vi "Structure Handler.vi"() -> ()   [LabVIEW 2010] (continued)
   .650136101028E-04   .693103789942E-04   .738911130024E-04   .787745775169E-04   .839807778292E-04\n   .895310410335E-04   .954481033336E-04   .101756203113E-03   .108481180149E-03   .115650581371E-03\n   .123293773602E-03   .131442063738E-03   .140128826854E-03   .149389642765E-03   .159262441590E-03\n   .169787658919E-03   .181008401214E-03   .192970622109E-03   .205723310339E-03   .219318690051E-03\n   .233812434316E-03   .249263892711E-03   .265736333886E-03   .283297204114E-03   .302018402857E-03\n   .321976576476E-03   .343253431267E-03   .365936067091E-03   .390117332948E-03   .415896205926E-03\n   .443378195057E-03   .472675771709E-03   .503908828239E-03   .537205166754E-03   .572701019950E-03\n   .610541606096E-03   .650881720414E-03   .693886365185E-03   .739731421127E-03   .788604362696E-03\n   .840705020160E-03   .896246391477E-03   .955455507177E-03   .101857435167E-02   .108586084462E-02\n   .115758988621E-02   .123405447041E-02   .131556687066E-02   .140245990241E-02   .149508826758E-02\n   .159382998615E-02   .169908792015E-02   .181129139623E-02   .193089793270E-02   .205839507779E-02\n   .219430236596E-02   .233917339963E-02   .249359806416E-02   .265820488411E-02   .283366352974E-02\n   .302068748250E-02   .322003686958E-02   .343252147732E-02   .365900395451E-02   .390040321649E-02\n   .415769806226E-02   .443193101665E-02   .472421241091E-02   .503572471499E-02   .536772713610E-02\n   .572156049811E-02   .609865241743E-02   .650052279140E-02   .692878961584E-02   .738517514896E-02\n   .787151243951E-02   .838975223731E-02   .894197030486E-02   .953037514915E-02   .101573161929E-01\n   .108252924048E-01   .115369614078E-01   .122951490860E-01   .131028597072E-01   .139632865812E-01\n   .148798232710E-01   .158560753728E-01   .168958728802E-01   .180032831452E-01   .191826244469E-01\n   .204384801745E-01   .217757136292E-01   .231994834433E-01   .247152596108E-01   .263288401171E-01\n   .280463681475E-01   .298743498448E-01   .318196725793E-01   .338896236775E-01   .360919095467E-01\n   .384346751137E-01   .409265234803E-01   .435765356742E-01   .463942903543E-01   .493898832987E-01\n   .525739464755E-01   .559576664626E-01   .595528019418E-01   .633716999509E-01   .674273105302E-01\n   .717331993426E-01   .763035577917E-01   .811532100904E-01   .862976166680E-01   .917528732159E-01\n   .975357045937E-01   .103663452719E+00   .110154057471E+00   .117026029513E+00   .124298413867E+00\n   .131990742895E+00   .140122977286E+00   .148715433467E+00   .157788695785E+00   .167363511634E+00\n   .177460667645E+00   .188100844913E+00   .199304451187E+00   .211091427879E+00   .223481029745E+00\n   .236491575107E+00   .250140164607E+00   .264442366603E+00   .279411867634E+00   .295060086708E+00\n   .311395752693E+00   .328424444740E+00   .346148096533E+00   .364564466156E+00   .383666574705E+00\n   .403442118234E+00   .423872859464E+00   .444934007698E+00   .466593597760E+00   .488811881305E+00\n   .511540746661E+00   .534723186242E+00   .558292833461E+00   .582173593824E+00   .606279397201E+00\n   .630514099889E+00   .654771565578E+00   .678935953260E+00   .702882236781E+00   .726476974553E+00\n   .749579338001E+00   .772042392823E+00   .793714607160E+00   .814441534495E+00   .834067585816E+00\n   .852437765062E+00   .869399194191E+00   .884802200660E+00   .898500682856E+00   .910351412094E+00\n   .920211879383E+00   .927936259976E+00   .933369060769E+00   .936336050196E+00   .936632166367E+00\n   .934006278440E+00   .928139957090E+00   .918838625658E+00\n ae wavefunction\n  -.102472886728E-04  -.108350209538E-04  -.114549459033E-04  -.121089170600E-04  -.127988910547E-04\n  -.135269336247E-04  -.142952259721E-04  -.151060714864E-04  -.159619028513E-04  -.168652895618E-04\n  -.178189458735E-04  -.188257392112E-04  -.198886990647E-04  -.210110264001E-04  -.221961036178E-04\n  -.234475050907E-04  -.247690083160E-04  -.261646057188E-04  -.276385171457E-04  -.291952030898E-04\n  -.308393786910E-04  -.325760285591E-04  -.344104224659E-04  -.363481319629E-04  -.383950479748E-04\n  -.405573994319E-04  -.428417730001E-04  -.452551339748E-04  -.478048484101E-04  -.504987065540E-04\n  -.533449476693E-04  -.563522863230E-04  -.595299402297E-04  -.628876597445E-04  -.664357590997E-04\n  -.701851494929E-04  -.741473741334E-04  -.783346453645E-04  -.827598839848E-04  -.874367608981E-04\n  -.923797412302E-04  -.976041310583E-04  -.103126126907E-03  -.108962868173E-03  -.115132492655E-03\n  -.121654195365E-03  -.128548290813E-03  -.135836278984E-03  -.143540915196E-03  -.151686284087E-03\n  -.160297877962E-03  -.169402679755E-03  -.179029250867E-03  -.189207824171E-03  -.199970402465E-03\n  -.211350862705E-03  -.223385066326E-03  -.236110976007E-03  -.249568779248E-03  -.263801019132E-03\n  -.278852732676E-03  -.294771597198E-03  -.311608085140E-03  -.329415627815E-03  -.348250788556E-03\n  -.368173445798E-03  -.389246986603E-03  -.411538511212E-03  -.435119049195E-03  -.460063787817E-03\n  -.486452313252E-03  -.514368865329E-03  -.543902606477E-03  -.575147905623E-03  -.608204637764E-03\n  -.643178500018E-03  -.680181344946E-03  -.719331531999E-03  -.760754297934E-03  -.804582147123E-03\n  -.850955262651E-03  -.900021939173E-03  -.951939038487E-03  -.100687246884E-02  -.106499768896E-02\n  -.112650023789E-02  -.119157629169E-02  -.126043324797E-02  -.133329033948E-02  -.141037927781E-02\n  -.149194492818E-02  -.157824601651E-02  -.166955586987E-02  -.176616319118E-02  -.186837286943E-02\n  -.197650682617E-02  -.209090489935E-02  -.221192576536E-02  -.233994790000E-02  -.247537057913E-02\n  -.261861491967E-02  -.277012496121E-02  -.293036878884E-02  -.309983969707E-02  -.327905739499E-02\n  -.346856925230E-02  -.366895158573E-02  -.388081098494E-02  -.410478567693E-02  -.434154692721E-02\n  -.459180047599E-02  -.485628800693E-02  -.513578864552E-02  -.543112048365E-02  -.574314212629E-02\n  -.607275425537E-02  -.642090120550E-02  -.678857254485E-02  -.717680465403E-02  -.758668229464E-02\n  -.801934015783E-02  -.847596438244E-02  -.895779403056E-02  -.946612250719E-02  -.100022989091E-01\n  -.105677292859E-01  -.111638777959E-01  -.117922677347E-01  -.124544824164E-01  -.131521658802E-01\n  -.138870233978E-01  -.146608217502E-01  -.154753892431E-01  -.163326154249E-01  -.172344504697E-01\n  -.181829041838E-01  -.191800445922E-01  -.202279960556E-01  -.213289368677E-01  -.224850962776E-01\n  -.236987508768E-01  -.249722202903E-01  -.263078621027E-01  -.277080659502E-01  -.291752467024E-01\n  -.307118366560E-01  -.323202766578E-01  -.340030060703E-01  -.357624514904E-01  -.376010141285E-01\n  -.395210557524E-01  -.415248830978E-01  -.436147306457E-01  -.457927416672E-01  -.480609474327E-01\n  -.504212444884E-01  -.528753698999E-01  -.554248743698E-01  -.580710931391E-01  -.608151145893E-01\n  -.636577464720E-01  -.665994797002E-01  -.696404496533E-01  -.727803949601E-01  -.760186137451E-01\n  -.793539173445E-01  -.827845815260E-01  -.863082952746E-01  -.899221072416E-01  -.936223699944E-01\n  -.974046822452E-01  -.101263829289E+00  -.105193721933E+00  -.109187334262E+00  -.113236640640E+00\n  -.117332552425E+00  -.121464854938E+00  -.125622145291E+00  -.129791771755E+00  -.133959775402E+00\n  -.138110834814E+00  -.142228214722E+00  -.146293719478E+00  -.150287652379E+00  -.154188781955E+00\n  -.157974316537E+00  -.161619888588E+00  -.165099550597E+00  -.168385784509E+00  -.171449526912E+00\n  -.174260212293E+00  -.176785836695E+00  -.178993044052E+00  -.180847237296E+00  -.182312716182E+00\n  -.183352843504E+00  -.183930241176E+00  -.184007017455E+00  -.183545026421E+00  -.182506160678E+00\n  -.180852678087E+00  -.178547563044E+00  -.175554922526E+00  -.171840416688E+00  -.167371723309E+00\n  -.162119034827E+00  -.156055586067E+00  -.149158210059E+00  -.141407918546E+00  -.132790502958E+00\n  -.123297150652E+00  -.112925070301E+00  -.101678119247E+00  -.895674246251E-01  -.766119890217E-01\n  -.628392704161E-01  -.482857252105E-01  -.329973022932E-01  -.170298753267E-01  -.449599868019E-03\n   .166668184700E-01   .342319587058E-01   .521476355883E-01   .703049796943E-01   .885846572927E-01\n   .106857238053E+00   .124983715590E+00   .142816183462E+00   .160198669259E+00   .176968132946E+00\n   .192955642537E+00   .207987747188E+00   .221888068880E+00   .234479122199E+00   .245584347951E+00\n   .255030323450E+00   .262649105328E+00   .268280669487E+00   .271775423505E+00   .272996768417E+00\n   .271823680061E+00   .268153271721E+00   .261903294683E+00   .253014532452E+00   .241453045815E+00\n   .227212227558E+00   .210314626215E+00   .190813497605E+00   .168794041580E+00   .144374279974E+00\n   .117705531020E+00   .889724362620E-01   .583924991851E-01   .262151011350E-01  -.728003019462E-02\n  -.417849123944E-01  -.769659613191E-01  -.112467199941E+00  -.147914017773E+00  -.182917473950E+00\n  -.217079101945E+00  -.249996050169E+00  -.281266155697E+00  -.310492338804E+00  -.337285915132E+00\n  -.361269394558E+00  -.382080559387E+00  -.399379300172E+00  -.412856108186E+00  -.422239455056E+00\n  -.427300826220E+00  -.427858101849E+00  -.423778169793E+00  -.414979071649E+00  -.401431580845E+00\n  -.383159989479E+00  -.360241927552E+00  -.332807157172E+00  -.301035398222E+00  -.265153310634E+00\n  -.225430782988E+00  -.182176673402E+00  -.135734133840E+00  -.864756317344E-01  -.347977671865E-01\n   .188840279327E-01   .741408308910E-01   .130535535272E+00   .187628052492E+00   .244980336901E+00\n   .302161166898E+00   .358750621194E+00   .414344200377E+00   .468556552153E+00   .521024757194E+00\n   .571411110889E+00   .619405293638E+00   .664725784944E+00   .707120394973E+00   .746365921412E+00\n   .782267188776E+00   .814655980838E+00   .843390443892E+00   .868355317176E+00   .889462932201E+00\n   .906654594240E+00   .919901848226E+00   .929207271714E+00   .934604632164E+00   .936158407443E+00\n   .933962745894E+00   .928139957090E+00   .918838625658E+00\n pseudo wavefunction\n   .352991027465E-09   .376321051042E-09   .401193011816E-09   .427708820114E-09   .455977121757E-09\n   .486113743230E-09   .518242166268E-09   .552494033810E-09   .589009689389E-09   .627938752181E-09\n   .669440730049E-09   .713685673115E-09   .760854870518E-09   .811141593229E-09   .864751885963E-09\n   .921905411418E-09   .982836350330E-09   .104779436099E-08   .111704560222E-08   .119087382390E-08\n   .126958152960E-08   .135349121612E-08   .144294669479E-08   .153831450029E-08   .163998539244E-08\n   .174837595728E-08   .186393031406E-08   .198712193490E-08   .211845558482E-08   .225846938996E-08\n   .240773704251E-08   .256687015132E-08   .273652074794E-08   .291738395820E-08   .311020085049E-08\n   .331576147212E-08   .353490808652E-08   .376853862430E-08   .401761036242E-08   .428314384652E-08\n   .456622707253E-08   .486801994458E-08   .518975902758E-08   .553276261393E-08   .589843612507E-08\n   .628827787002E-08   .670388518454E-08   .714696097604E-08   .761932070107E-08   .812289980387E-08\n   .865976164672E-08   .923210596427E-08   .984227787670E-08   .104927774986E-07   .111862701828E-07\n   .119255974416E-07   .127137885890E-07   .135540731535E-07   .144498941103E-07   .154049219889E-07\n   .164230699118E-07   .175085096291E-07   .186656886107E-07   .198993482698E-07   .212145433901E-07\n   .226166628369E-07   .241114516374E-07   .257050345200E-07   .274039410095E-07   .292151321810E-07\n   .311460291817E-07   .332045436377E-07   .353991100712E-07   .377387204590E-07   .402329610758E-07\n   .428920517725E-07   .457268878502E-07   .487490847013E-07   .519710254020E-07   .554059114492E-07\n   .590678168511E-07   .629717457928E-07   .671336941124E-07   .715707148406E-07   .763009880718E-07\n   .813438954526E-07   .867200995936E-07   .924516287288E-07   .985619669711E-07   .105076150532E-06\n   .112020870298E-06   .119424581195E-06   .127317618764E-06   .135732323461E-06   .144703173155E-06\n   .154266924388E-06   .164462762979E-06   .175332464561E-06   .186920565753E-06   .199274546618E-06\n   .212445025198E-06   .226485964898E-06   .241454895568E-06   .257413149209E-06   .274426111244E-06\n   .292563488397E-06   .311899594272E-06   .332513653809E-06   .354490127851E-06   .377919059166E-06\n   .402896441323E-06   .429524611954E-06   .457912671992E-06   .488176932618E-06   .520441391731E-06\n   .554838241911E-06   .591508411929E-06   .630602144051E-06   .672279609474E-06   .716711564420E-06\n   .764080049586E-06   .814579135792E-06   .868415718892E-06   .925810367198E-06   .986998224881E-06\n   .105222997505E-05   .112177286643E-05   .119591180790E-05   .127495053523E-05   .135921285499E-05\n   .144904397052E-05   .154481189552E-05   .164690896091E-05   .175575342131E-05   .187179116750E-05\n   .199549755192E-05   .212737933479E-05   .226797675859E-05   .241786575958E-05   .257766032513E-05\n   .274801500683E-05   .292962759922E-05   .312324199548E-05   .332965123134E-05   .354970072992E-05\n   .378429176054E-05   .403438512567E-05   .430100509096E-05   .458524357445E-05   .488826461184E-05\n   .521130911618E-05   .555569995111E-05   .592284733843E-05   .631425462178E-05   .673152440997E-05\n   .717636512477E-05   .765059797966E-05   .815616441788E-05   .869513403977E-05   .926971305144E-05\n   .988225326896E-05   .105352617143E-04   .112314108416E-04   .119735494351E-04   .127647142226E-04\n   .136081422505E-04   .145072840707E-04   .154658177921E-04   .164876640517E-04   .175770019673E-04\n   .187382861324E-04   .199762647237E-04   .212959987912E-04   .227028828071E-04   .242026665564E-04\n   .258014784535E-04   .275058503770E-04   .293227441208E-04   .312595795632E-04   .333242646647E-04\n   .355252274107E-04   .378714498215E-04   .403725041624E-04   .430385914897E-04   .458805826821E-04\n   .489100621118E-04   .521393741199E-04   .555816724705E-04   .592509729684E-04   .631622094336E-04\n   .673312932398E-04   .717751766317E-04   .765119200529E-04   .815607637215E-04   .869422037107E-04\n   .926780727984E-04   .987916263670E-04   .105307633647E-03   .112252474613E-03   .119654242849E-03\n   .127542854732E-03   .135950165266E-03   .144910090943E-03   .154458740012E-03   .164634550536E-03\n   .175478436648E-03   .187033943428E-03   .199347410807E-03   .212468146962E-03   .226448611615E-03\n   .241344609707E-03   .257215495864E-03   .274124390140E-03   .292138405428E-03   .311328887000E-03\n   .331771664562E-03   .353547317209E-03   .376741451614E-03   .401444993766E-03   .427754494472E-03\n   .455772448807E-03   .485607629577E-03   .517375434769E-03   .551198248816E-03   .587205817364E-03\n   .625535635033E-03   .666333345435E-03   .709753152467E-03   .755958241591E-03   .805121209423E-03\n   .857424499599E-03   .913060842326E-03   .972233694523E-03   .103515767678E-02   .110205900260E-02\n   .117317589457E-02   .124875898098E-02   .132907166554E-02   .141439046110E-02   .150500527724E-02\n   .160121964948E-02   .170335089620E-02   .181173018683E-02   .192670250258E-02   .204862646782E-02\n   .217787402718E-02   .231482993932E-02   .245989105447E-02   .261346533761E-02   .277597059411E-02\n   .294783284795E-02   .312948431631E-02   .332136091583E-02   .352389922746E-02   .373753283668E-02\n   .396268795459E-02   .419977821319E-02   .444919851374E-02   .471131779174E-02   .498647054434E-02\n   .527494694670E-02   .557698136200E-02   .589273902574E-02   .622230065848E-02   .656564473144E-02\n   .692262707728E-02   .729295750228E-02   .767617301739E-02   .807160726257E-02   .847835565252E-02\n   .889523572126E-02   .932074208875E-02   .975299541408E-02   .101896846375E-01   .106280017477E-01\n   .110645682410E-01   .114953523684E-01   .119155761909E-01   .123196113926E-01   .127008627264E-01\n   .130516379023E-01   .133630026652E-01   .136246197664E-01   .138245705014E-01   .139491574888E-01\n   .139826874030E-01   .139072324662E-01   .137023696688E-01   .133448969538E-01   .128085259919E-01\n   .120635517471E-01   .110764998264E-01   .980975371236E-02   .822116546231E-02   .626365546011E-02\n   .388480945228E-02   .102648457808E-02  -.237555937194E-02  -.639198140091E-02  -.111001039357E-01\n  -.165840417070E-01  -.229346641739E-01  -.302493262711E-01  -.386312846112E-01  -.481886952189E-01\n  -.590330642855E-01  -.712769955167E-01  -.850310471077E-01  -.100399479677E+00  -.117474646201E+00\n  -.136329750145E+00  -.157003219319E+00  -.179549174600E+00\n ae wavefunction\n   .137618411224E-07   .145510584709E-07   .153835077169E-07   .162616777311E-07   .171881958183E-07\n   .181658357929E-07   .191975265164E-07   .202863609227E-07   .214356055619E-07   .226487106923E-07\n   .239293209542E-07   .252812866604E-07   .267086757403E-07   .282157863766E-07   .298071603760E-07\n   .314875973191E-07   .332621695339E-07   .351362379449E-07   .371154688484E-07   .392058516699E-07\n   .414137177637E-07   .437457603151E-07   .462090554122E-07   .488110843581E-07   .515597572965E-07\n   .544634382289E-07   .575309715088E-07   .607717098976E-07   .641955442797E-07   .678129351313E-07\n   .716349458512E-07   .756732780630E-07   .799403090046E-07   .844491311339E-07   .892135940765E-07\n   .942483490595E-07   .995688959770E-07   .105191633244E-06   .111133910604E-06   .117414085065E-06\n   .124051580151E-06   .131066948660E-06   .138481939147E-06   .146319566334E-06   .154604185695E-06\n   .163361572454E-06   .172619005255E-06   .182405354776E-06   .192751177583E-06   .203688815521E-06\n   .215252500969E-06   .227478468301E-06   .240405071901E-06   .254072911129E-06   .268524962617E-06\n   .283806720325E-06   .299966343805E-06   .317054815127E-06   .335126104962E-06   .354237348345E-06\n   .374449030652E-06   .395825184360E-06   .418433597199E-06   .442346032313E-06   .467638461093E-06\n   .494391309384E-06   .522689717766E-06   .552623816695E-06   .584289017276E-06   .617786318510E-06\n   .653222631875E-06   .690711124149E-06   .730371579412E-06   .772330781220E-06   .816722915955E-06\n   .863689998438E-06   .913382320884E-06   .965958926355E-06   .102158810790E-05   .108044793458E-05\n   .114272680570E-05   .120862403447E-05   .127835046250E-05   .135212910649E-05   .143019583852E-05\n   .151280010133E-05   .160020566023E-05   .169269139287E-05   .179055211860E-05   .189409946893E-05\n   .200366280045E-05   .211959015197E-05   .224224924727E-05   .237202854503E-05   .250933833742E-05\n   .265461189882E-05   .280830668601E-05   .297090559128E-05   .314291824958E-05   .332488240099E-05\n   .351736530945E-05   .372096523867E-05   .393631298599E-05   .416407347460E-05   .440494740451E-05\n   .465967296228E-05   .492902758925E-05   .521382980755E-05   .551494110318E-05   .583326786436E-05\n   .616976337358E-05   .652542985073E-05   .690132054423E-05   .729854186664E-05   .771825557003E-05\n   .816168095601E-05   .863009711419E-05   .912484518192E-05   .964733061696E-05   .101990254738E-04\n   .107814706729E-04   .113962782501E-04   .120451335740E-04   .127297975143E-04   .134521085448E-04\n   .142139847628E-04   .150174258019E-04   .158645146168E-04   .167574191139E-04   .176983935982E-04\n   .186897800086E-04   .197340089040E-04   .208336001672E-04   .219911633850E-04   .232093978605E-04\n   .244910922131E-04   .258391235149E-04   .272564559089E-04   .287461386529E-04   .303113035259E-04\n   .319551615320E-04   .336809988326E-04   .354921718317E-04   .373921013383E-04   .393842657226E-04\n   .414721929817E-04   .436594516248E-04   .459496402860E-04   .483463759690E-04   .508532808261E-04\n   .534739673698E-04   .562120220180E-04   .590709868685E-04   .620543396013E-04   .651654714088E-04\n   .684076628539E-04   .717840575626E-04   .752976336611E-04   .789511728733E-04   .827472272074E-04\n   .866880831647E-04   .907757234225E-04   .950117859542E-04   .993975205696E-04   .103933742878E-03\n   .108620785699E-03   .113458447978E-03   .118445941286E-03   .123581834014E-03   .128863993431E-03\n   .134289525781E-03   .139854714662E-03   .145554957975E-03   .151384703761E-03   .157337385325E-03\n   .163405356054E-03   .169579824419E-03   .175850789667E-03   .182206978733E-03   .188635784929E-03\n   .195123208948E-03   .201653802707E-03   .208210616552E-03   .214775150314E-03   .221327308779E-03\n   .227845362183E-03   .234305912539E-03   .240683866744E-03   .246952417629E-03   .253083034207E-03\n   .259045462384E-03   .264807737263E-03   .270336207888E-03   .275595574924E-03   .280548941304E-03\n   .285157875379E-03   .289382485651E-03   .293181505721E-03   .296512387798E-03   .299331402794E-03\n   .301593744846E-03   .303253637785E-03   .304264440783E-03   .304578750103E-03   .304148493556E-03\n   .302925014008E-03   .300859138086E-03   .297901226081E-03   .294001199062E-03   .289108539236E-03\n   .283172259918E-03   .276140841838E-03   .267962133199E-03   .258583211806E-03   .247950208792E-03\n   .236008095016E-03   .222700433166E-03   .207969100890E-03   .191753993121E-03   .173992714884E-03\n   .154620279546E-03   .133568831453E-03   .110767416410E-03   .861418285720E-04   .596145684637E-04\n   .311049544574E-04   .529439242712E-06  -.321978070211E-04  -.671639762186E-04  -.104456289332E-03\n  -.144160179057E-03  -.186356927478E-03  -.231120713144E-03  -.278515028872E-03  -.328588420472E-03\n  -.381369473043E-03  -.436860957449E-03  -.495033060545E-03  -.555815651377E-03  -.619089564699E-03\n  -.684676904215E-03  -.752330385191E-03  -.821721758001E-03  -.892429386495E-03  -.963925098327E-03\n  -.103556047622E-02  -.110655281599E-02  -.117597103657E-02  -.124272188717E-02  -.130553685406E-02\n  -.136296022244E-02  -.141333879453E-02  -.145481380079E-02  -.148531556965E-02  -.150256154443E-02\n  -.150405826431E-02  -.148710796411E-02  -.144882049000E-02  -.138613123116E-02  -.129582564182E-02\n  -.117457056618E-02  -.101895203840E-02  -.825519036647E-03  -.590833860362E-03  -.311532762146E-03\n   .155972077532E-04   .393522461006E-03   .824854923326E-03   .131174286271E-02   .185576281993E-02\n   .245780651869E-02   .311795882336E-02   .383536809019E-02   .460811220956E-02   .543306302164E-02\n   .630575035283E-02   .722022568213E-02   .816892493328E-02   .914253008746E-02   .101298298504E-01\n   .111175801652E-01   .120903657699E-01   .130304642481E-01   .139177141349E-01   .147293886237E-01\n   .154400763014E-01   .160215701253E-01   .164427655922E-01   .166695688056E-01   .166648149728E-01\n   .163881978477E-01   .157962106791E-01   .148420993614E-01   .134758283310E-01   .116440594656E-01\n   .929014402068E-02   .635412837335E-02   .277277742664E-02  -.152037455845E-02  -.659492918765E-02\n  -.125234665193E-01  -.193813145676E-01  -.272462537562E-01  -.361981844009E-01  -.463187934547E-01\n  -.576912499803E-01  -.703999444832E-01  -.845302751275E-01  -.100168480149E+00  -.117401518650E+00\n  -.136317006642E+00  -.157003219319E+00  -.179549174600E+00\n pseudo wavefunction\n   .177267231484E-12   .195128511823E-12   .214789478054E-12   .236431464844E-12   .260254077969E-12\n   .286477035300E-12   .315342193273E-12   .347115777552E-12   .382090838451E-12   .420589953759E-12\n   .462968203902E-12   .509616446875E-12   .560964923163E-12   .617487223878E-12   .679704658728E-12\n   .748191064104E-12   .823578095610E-12   .906561053883E-12   .997905297400E-12   .109845330144E-11\n   .120913242831E-11   .133096348048E-11   .146507011550E-11   .161268920963E-11   .177518226563E-11\n   .195404796997E-11   .215093601541E-11   .236766231619E-11   .260622575638E-11   .286882662574E-11\n   .315788691318E-11   .347607264494E-11   .382631847360E-11   .421185474456E-11   .463623728985E-11\n   .510338022379E-11   .561759204322E-11   .618361536512E-11   .680667066813E-11   .749250444146E-11\n   .824744218521E-11   .907844675100E-11   .999318256090E-11   .110000862970E-10   .121084447137E-10\n   .133284802901E-10   .146714455128E-10   .161497266584E-10   .177769580336E-10   .195681477248E-10\n   .215398160195E-10   .237101477740E-10   .260991601340E-10   .287288871543E-10   .316235830205E-10\n   .348099457478E-10   .383173634188E-10   .421781852321E-10   .464280198620E-10   .511060638799E-10\n   .562554632679E-10   .619237113579E-10   .681630868661E-10   .750311360646E-10   .825912035356E-10\n   .909130164034E-10   .100073327434E-09   .110156622933E-09   .121255901970E-09   .133473534114E-09\n   .146922203605E-09   .161725948640E-09   .178021305397E-09   .195958567318E-09   .215703171276E-09\n   .237437223417E-09   .261361178744E-09   .287695689926E-09   .316683642404E-09   .348592394542E-09\n   .383716243503E-09   .422379139576E-09   .464937674003E-09   .511784367855E-09   .563351292293E-09\n   .620114053603E-09   .682596179765E-09   .751373949000E-09   .827081704849E-09   .910417706791E-09\n   .100215057037E-08   .110312635620E-08   .121427637332E-08   .133662576872E-08   .147130298242E-08\n   .161955015520E-08   .178273458500E-08   .196236133771E-08   .216008712857E-08   .237773560226E-08\n   .261731415265E-08   .288103243724E-08   .317132275718E-08   .349086249070E-08   .384259878701E-08\n   .422977574828E-08   .465596435055E-08   .512509537940E-08   .564149568430E-08   .620992808586E-08\n   .683563530424E-08   .752438831374E-08   .828253956965E-08   .911708159823E-08   .100357114903E-07\n   .110469018932E-07   .121599791561E-07   .133852093488E-07   .147338929490E-07   .162184690689E-07\n   .178526301847E-07   .196514484268E-07   .216315145940E-07   .238110911760E-07   .262102807946E-07\n   .288512116168E-07   .317582414515E-07   .349581824108E-07   .384805482090E-07   .423578263805E-07\n   .466257779270E-07   .513237671579E-07   .564951247679E-07   .621875474984E-07   .684535380719E-07\n   .753508894551E-07   .829432179206E-07   .913005498212E-07   .100499967493E-06   .110626320242E-06\n   .121773006977E-06   .134042837705E-06   .147548981841E-06   .162416012071E-06   .178781053415E-06\n   .196795048071E-06   .216624147728E-06   .238451246178E-06   .262477666373E-06   .288925017504E-06\n   .318037239210E-06   .350082851806E-06   .385357433274E-06   .424186345884E-06   .466927737604E-06\n   .513975845980E-06   .565764635006E-06   .622771798513E-06   .685523167052E-06   .754597558918E-06\n   .830632120119E-06   .914328202545E-06   .100645783462E-05   .110787084417E-05   .121950269922E-05\n   .134238313919E-05   .147764567611E-05   .162653805357E-05   .179043376008E-05   .197084470305E-05\n   .216943516055E-05   .238803713959E-05   .262866728293E-05   .289354548047E-05   .318511535733E-05\n   .350606682774E-05   .385936092342E-05   .424825712563E-05   .467634345389E-05   .514756958921E-05\n   .566628333836E-05   .623727077631E-05   .686580043820E-05   .755767196958E-05   .831926968534E-05\n   .915762153277E-05   .100804640049E-04   .110963136049E-04   .122145455239E-04   .134454802607E-04\n   .148004789865E-04   .162920485386E-04   .179339570169E-04   .197413610551E-04   .217309459486E-04\n   .239210799391E-04   .263319840901E-04   .289859193303E-04   .319073924057E-04   .351233826543E-04\n   .386635917151E-04   .425607184965E-04   .468507619657E-04   .515733545831E-04   .567721294918E-04\n   .624951248914E-04   .687952293743E-04   .757306723900E-04   .833655644268E-04   .917704919735E-04\n   .101023172839E-03   .111209177984E-03   .122422726642E-03   .134767562225E-03   .148357917245E-03\n   .163319576369E-03   .179791047642E-03   .197924852956E-03   .217888949984E-03   .239868299087E-03\n   .264066590060E-03   .290708145179E-03   .320040016680E-03   .352334298733E-03   .387890676023E-03\n   .427039233419E-03   .470143553721E-03   .517604133365E-03   .569862149064E-03   .627403611879E-03\n   .690763949034E-03   .760533058090E-03   .837360882811E-03   .921963565285E-03   .101513023470E-02\n   .111773049960E-02   .123072271762E-02   .135516312450E-02   .149221591326E-02   .164316436368E-02\n   .180942313350E-02   .199255183450E-02   .219427002978E-02   .241647380359E-02   .266125407099E-02\n   .293091681294E-02   .322800544219E-02   .355532552753E-02   .391597212840E-02   .431336001852E-02\n   .475125710724E-02   .523382139980E-02   .576564187362E-02   .635178368709E-02   .699783818060E-02\n   .770997817641E-02   .849501913505E-02   .936048678149E-02   .103146918737E-01   .113668128506E-01\n   .125269871635E-01   .138064121687E-01   .152174565314E-01   .167737831718E-01   .184904848583E-01\n   .203842336354E-01   .224734453453E-01   .247784605712E-01   .273217433915E-01   .301280993745E-01\n   .332249142671E-01   .366424148226E-01   .404139531638E-01   .445763159812E-01   .491700596945E-01\n   .542398724605E-01   .598349635467E-01   .660094801087E-01   .728229507563E-01   .803407544570E-01\n   .886346122542E-01   .977830979381E-01   .107872162152E+00   .118995662400E+00   .131255889004E+00\n   .144764074182E+00   .159640868060E+00   .176016761568E+00   .194032431779E+00   .213838980399E+00\n   .235598030773E+00   .259481643242E+00   .285672002899E+00   .314360828291E+00   .345748444593E+00\n   .380042460821E+00   .417455988444E+00   .458205338955E+00   .502507141713E+00   .550574831420E+00\n   .602614468362E+00   .658819874780E+00   .719367098474E+00   .784408250325E+00   .854064805549E+00\n   .928420507861E+00   .100751406833E+01   .109133190169E+01   .117980118454E+01   .127278354258E+01\n   .137006966305E+01   .147137742340E+01   .157664611943E+01\n ae wavefunction\n   .535557091704E-08   .584615313749E-08   .637852560608E-08   .695650990210E-08   .758425806990E-08\n   .826628296378E-08   .900749126748E-08   .981321943576E-08   .106892728292E-07   .116419683371E-07\n   .126781808104E-07   .138053936581E-07   .150317539875E-07   .163661327113E-07   .178181900766E-07\n   .193984471166E-07   .211183635708E-07   .229904228708E-07   .250282248432E-07   .272465868411E-07\n   .296616540847E-07   .322910200607E-07   .351538579091E-07   .382710638186E-07   .416654135374E-07\n   .453617332187E-07   .493870859284E-07   .537709752675E-07   .585455677026E-07   .637459353389E-07\n   .694103210402E-07   .755804279757E-07   .823017358680E-07   .896238464348E-07   .976008607458E-07\n   .106291791475E-06   .115761013316E-06   .126078755115E-06   .137321637649E-06   .149573261301E-06\n   .162924848323E-06   .177475944810E-06   .193335187973E-06   .210621144868E-06   .229463229277E-06\n   .250002704098E-06   .272393777294E-06   .296804800206E-06   .323419577871E-06   .352438801904E-06\n   .384081617500E-06   .418587337205E-06   .456217315308E-06   .497256998019E-06   .542018166025E-06\n   .590841387595E-06   .644098702138E-06   .702196555972E-06   .765579014149E-06   .834731274431E-06\n   .910183511962E-06   .992515085916E-06   .108235914231E-05   .118040765045E-05   .128741691394E-05\n   .140421360120E-05   .153170134439E-05   .167086796061E-05   .182279335395E-05   .198865816282E-05\n   .216975322265E-05   .236748992100E-05   .258341152907E-05   .281920560166E-05   .307671754594E-05\n   .335796546920E-05   .366515642546E-05   .400070419254E-05   .436724872291E-05   .476767742530E-05\n   .520514844837E-05   .568311615361E-05   .620535898190E-05   .677600993702E-05   .739958992971E-05\n   .808104424844E-05   .882578244719E-05   .963972196691E-05   .105293358364E-04   .115017048293E-04\n   .125645744884E-04   .137264174648E-04   .149965016599E-04   .163849647036E-04   .179028953450E-04\n   .195624223894E-04   .213768118654E-04   .233605731714E-04   .255295750119E-04   .279011720082E-04\n   .304943429440E-04   .333298416879E-04   .364303619275E-04   .398207169443E-04   .435280357643E-04\n   .475819771328E-04   .520149628821E-04   .568624323930E-04   .621631199927E-04   .679593572815E-04\n   .742974025452E-04   .812277995842E-04   .888057684784E-04   .970916310060E-04   .106151273651E-03\n   .116056651362E-03   .126886335469E-03   .138726109423E-03   .151669616309E-03   .165819062365E-03\n   .181285981054E-03   .198192062573E-03   .216670054020E-03   .236864735810E-03   .258933980321E-03\n   .283049899139E-03   .309400085708E-03   .338188960618E-03   .369639227222E-03   .403993445736E-03\n   .441515734478E-03   .482493607363E-03   .527239957303E-03   .576095195662E-03   .629429558406E-03\n   .687645590114E-03   .751180817511E-03   .820510624648E-03   .896151342322E-03   .978663564752E-03\n   .106865570691E-02   .116678781619E-02   .127377565250E-02   .139039505069E-02   .151748657989E-02\n   .165596051352E-02   .180680212425E-02   .197107731740E-02   .214993861579E-02   .234463150841E-02\n   .255650117400E-02   .278699958957E-02   .303769303196E-02   .331026997863E-02   .360654941141E-02\n   .392848952388E-02   .427819682960E-02   .465793566447E-02   .507013807148E-02   .551741405100E-02\n   .600256215333E-02   .652858038310E-02   .709867737733E-02   .771628380971E-02   .838506396372E-02\n   .910892740586E-02   .989204067809E-02   .107388389144E-01   .116540372722E-01   .126426420512E-01\n   .137099613582E-01   .148616151513E-01   .161035444835E-01   .174420197380E-01   .188836476261E-01\n   .204353766962E-01   .221045010702E-01   .238986620996E-01   .258258475992E-01   .278943882806E-01\n   .301129509672E-01   .324905281293E-01   .350364232274E-01   .377602313017E-01   .406718142038E-01\n   .437812698306E-01   .470988947080E-01   .506351392801E-01   .544005552922E-01   .584057346980E-01\n   .626612395711E-01   .671775225433E-01   .719648373193E-01   .770331388378E-01   .823919726537E-01\n   .880503531153E-01   .940166299175E-01   .100298342637E+00   .106902062927E+00   .113833224167E+00\n   .121095938523E+00   .128692801551E+00   .136624684701E+00   .144890516314E+00   .153487051916E+00\n   .162408634982E+00   .171646949578E+00   .181190766703E+00   .191025686502E+00   .201133878922E+00\n   .211493825815E+00   .222080067897E+00   .232862960408E+00   .243808441743E+00   .254877819694E+00\n   .266027580335E+00   .277209224901E+00   .288369140290E+00   .299448509029E+00   .310383264646E+00\n   .321104098278E+00   .331536521915E+00   .341600992660E+00   .351213100691E+00   .360283821210E+00\n   .368719828095E+00   .376423865651E+00   .383295176394E+00   .389229988984E+00   .394122080847E+00\n   .397863441927E+00   .400345073211E+00   .401457947613E+00   .401094136245E+00   .399148068493E+00\n   .395517872662E+00   .390106751775E+00   .382824375227E+00   .373588286907E+00   .362325332199E+00\n   .348973096502E+00   .333481337937E+00   .315813392641E+00   .295947532026E+00   .273878254160E+00\n   .249617493172E+00   .223195730222E+00   .194662987245E+00   .164089681231E+00   .131567313019E+00\n   .972089612288E-01   .611495499793E-01   .235458591212E-01  -.154237513487E-01  -.555599253720E-01\n  -.966432190948E-01  -.138435344127E+00  -.180680758539E+00  -.223108628584E+00  -.265435190321E+00\n  -.307366500752E+00  -.348601411827E+00  -.388834295872E+00  -.427756778344E+00  -.465058000559E+00\n  -.500424206695E+00  -.533540096861E+00  -.564094053593E+00  -.591785950516E+00  -.616333933335E+00\n  -.637478529600E+00  -.654985045141E+00  -.668645509828E+00  -.678280660929E+00  -.683741885001E+00\n  -.684912828516E+00  -.681710402251E+00  -.674085030959E+00  -.662020139579E+00  -.645530959409E+00\n  -.624662775943E+00  -.599488740411E+00  -.570107351133E+00  -.536639690231E+00  -.499226481008E+00\n  -.458025014803E+00  -.413205983091E+00  -.364950242739E+00  -.313445539176E+00  -.258883212654E+00\n  -.201454915997E+00  -.141349372871E+00  -.787492042753E-01  -.138278434185E-01   .532534454775E-01\n   .122348422307E+00   .193328547557E+00   .266085373571E+00   .340532496791E+00   .416606938857E+00\n   .494269972861E+00   .573507668095E+00   .654331656637E+00   .736780660323E+00   .820923101590E+00\n   .906860813490E+00   .994733629756E+00   .108472460957E+01   .117706574281E+01   .127204411774E+01\n   .137000863656E+01   .147137742340E+01   .157664611943E+01\n End of Dataset\n"] -> [w685]
          shift-right: [w681] -> w674
          shift-left: "" -> [w680]
          tunnel: w675 -> [w679]
          n388 = Search 1D Array(1D array=w679, element=w684) -> (index of element=w683:i32)  [unwired: 1 in]
          n389 = Index Array(array=w685, index=w683) -> (element=w682:string)
          n390 = Concatenate Strings(w680, w682) -> (w681:string)
        }
        "POTCAR File" <- w674
      }
      event "Send Structure to DB": Value Change {
        n391 = event-data() -> ()  [unwired: 1 in, 5 out]
        n392 = local read "Database UDL"() -> (w690:path)
        n393 = call-poly <vilib>:"DB Tools Open Connection.vi"("connection information"=w690) -> ("connection reference"=w692:T17)  [unwired: 7 in, 1 out]
        n394 = call <vilib>:"Set Busy.vi"() -> ("error out"=w693:errorcluster)  [unwired: 10 in, 1 out]
        n395 = stacked-sequence {
          tunnel: w693 -> [w701]
          tunnel: [w698] -> w688
          tunnel: w692 -> [w717]
          tunnel: [w697] -> w691
          tunnel: [w696] -> w687
          frame #0 {
            n396 = local read "Current Atomic Structure"() -> (w718:T3)
            n397 = Unbundle By Name(w718) -> ("# of atoms"=w695:i32, "Lattice vector a"=w713:dbl[], "Lattice vector b"=w715:dbl[], "Lattice vector c"=w714:dbl[], "Atoms Array"=w702:T20)  [unwired: 1 out]
            n398 = Build Array(w713, w715, w714) -> (w716:dbl[][])
            n399 = Build Array(w715, w714, w713) -> (w712:dbl[][])
            n400 = for {
              tunnel: w716 -> [w749] mode=indexing
              tunnel: w712 -> [w748] mode=indexing
              tunnel: [w744] -> w711 mode=indexing
              tunnel: [w740] -> w710 mode=indexing
              n401 = call-poly <vilib>:"Vector Norm.vi"("Input Vector"=w749) -> ("norm"=w744:dbl)  [unwired: 9 in, 1 out]
              n402 = call-poly <vilib>:"Dot Product.vi"("Y Vector"=w748, "X Vector"=w749) -> ("X * Y"=w750:dbl)  [unwired: 1 out]
              n403 = call-poly <vilib>:"Vector Norm.vi"("Input Vector"=w748) -> ("norm"=w747:dbl)  [unwired: 9 in, 1 out]
              n404 = Multiply(x=w744, y=w747) -> (x*y=w746:dbl)
              n405 = Divide(x=w750, y=w746) -> (x/y=w745:dbl)
              n406 = Inverse Cosine(1:w745) -> (0:w741:dbl)
              n407 = Divide(x=360.0, y=6.283185307179586) -> (x/y=w742:dbl)
              n408 = Multiply(x=w742, y=w741) -> (x*y=w740:dbl)
            }
            n409 = Build Array (concatenate)(w711, w710, w713, w715, w714) -> (w709:dbl[])
            n410 = Number To Decimal String(number=w695) -> (decimal integer string=w694:string)  [unwired: 1 in]
            n411 = local read "Structure Name"() -> (w703:string)
            n412 = local read "Structure ID"() -> (w696:string)
            n413 = Number To Exponential String(number=w709, precision (6)=i16 12) -> (E-format string=w707:string[])  [unwired: 2 in]
            n414 = Build Array (concatenate)(w696, w703, w694, w707) -> (w706:string[])
            n415 = Array To Cluster(array=w706) -> (cluster=w705:T25)
            n416 = call <vilib>:"DB Tools Insert Data.vi"("data"=w705, "error in (no error)"=w701, "table"="Structure_Summary", "connection reference"=w717) -> ("error out"=w700:errorcluster, "connection reference out"=w699:T17)  [unwired: 6 in]
            n417 = for {
              tunnel: w702 -> [w726] mode=indexing
              shift-right: [w723] -> w698
              shift-left: w700 -> [w724]
              shift-right: [w722] -> w697
              shift-left: w699 -> [w725]
              tunnel: w696 -> [w719]
              n418 = Unbundle By Name(w726) -> ("Atom Name"=w721:string, "Positions (Direct)"=w720:dbl[][])
              n419 = for {
                shift-right: [w737] -> w722
                shift-left: w725 -> [w738]
                shift-right: [w735] -> w723
                shift-left: w724 -> [w736]
                tunnel: w721 -> [w734]
                tunnel: w720 -> [w732] mode=indexing
                tunnel: w719 -> [w733]
                n420 = Index Array(array=w732) -> (element #1=w731:dbl, element #2=w730:dbl, element #3=w729:dbl)  [unwired: 3 in]
                n421 = Bundle("Structure ID"=w733, "Atom Name"=w734, "Numeric"=w731, "Numeric"=w730, "Numeric"=w729) -> (w728:T26)  [unwired: 1 in]
                n422 = call <vilib>:"DB Tools Insert Data.vi"("data"=w728, "error in (no error)"=w736, "table"="Structure_Atoms", "connection reference"=w738) -> ("error out"=w735:errorcluster, "connection reference out"=w737:T17)  [unwired: 6 in]
              }
            }
          }
        }
        n423 = call <vilib>:"DB Tools Close Connection.vi"("error in (no error)"=w688, "connection reference"=w691) -> ("error out"=w689:errorcluster)  [unwired: 5 in]
        n424 = call <vilib>:"Unset Busy.vi"("error in (no error)"=w688) -> ("error out"=w686:errorcluster)  [unwired: 10 in]
        n425 = property on="Structure ID" class="Str"(error in=w686, "Val(Sgnl)"=w687) -> ()  [unwired: 1 in, 2 out]
        n426 = call <vilib>:"General Error Handler.vi"("error in (no error)"=w689) -> ()  [unwired: 10 in, 5 out]
      }
      event "Structure ID", "Structure Name": Value Change {
        n427 = event-data() -> ()  [unwired: 1 in, 5 out]
        n428 = local read "Structure ID"() -> (w761:string)
        n429 = call-poly <vilib>:"DB Tools Open Connection.vi"("connection information"="Database UDL") -> ("error out"=w764:errorcluster, "connection reference"=w772:T17)  [unwired: 7 in]
        n430 = Concatenate Strings("WHERE Structure_ID = '", w761, "'" ("string")) -> (w768:string)
        n431 = call <vilib>:"DB Tools Select Data.vi"("condition"=w768, "error in (no error)"=w764, "table"="Structure_Summary", "connection reference"=w772) -> ("error out"=w765:errorcluster, "data"=w759:variant[][], "connection reference out"=w766:T17)  [unwired: 2 in]
        n432 = Empty Array?(array=w759) -> (empty?=w767:bool)
        n433 = call <vilib>:"DB Tools Close Connection.vi"("error in (no error)"=w765, "connection reference"=w766) -> ("error out"=w757:errorcluster)  [unwired: 5 in]
        n434 = call <vilib>:"Clear Errors.vi"("error in (no error)"=w757) -> ()  [unwired: 6 in, 1 out]
        n435 = Not(x=w767) -> (.not. x?=w760:bool)
        "Exists?" <- w760
        n436 = disable-structure shown="Enabled" {
          disable-tunnel: w760 -> [w777 _]
          disable-tunnel: w759 -> [w776 _]
          disable-tunnel: "Structure Name" -> [w775 w817]
          disable-tunnel: [w774 w817] -> w756
          frame Disabled {
            n437 = case shown="True" w777 {
              tunnel: w776 -> [_ w784]
              tunnel: [w778 w779] -> w774
              tunnel: w775 -> [w778 _]
              frame False {
              }
              frame True {
                n438 = Index Array(array=w784, index (row)=0, index (col)=1 ("disabled index (col)")) -> (element=w781:variant)
                n439 = xnode "Database Variant To Data"("database variant"=w781, "type"="") -> ("data"=w779:string)  [unwired: 1 in, 1 out]
                n440 = local write "Structure Name"(w779) -> ()
              }
            }
          }
          frame Enabled {
          }
        }
        n441 = local read "Current Atomic Structure"() -> (w763:T3)
        n442 = Bundle By Name(cluster=w763, "Structure Name"=w756) -> (w762:T3)
        n443 = call <vilib>:"Search and Replace Pattern.vi"("string"=w756, "regular expression (\"\")"="[\\s()\\[\\]]" ("regular expression (\"\")"), "replace string (\"\")"="_" ("replace string (\"\")"), "replace all? (F)"=TRUE) -> ("result string"=w754:string)  [unwired: 1 in, 1 out]
        n444 = local write "Current Atomic Structure"(w762) -> ()
        n445 = call <vilib>:"Trim Whitespace.vi"("string"=w754) -> ("trimmed string"=w753:string)  [unwired: 1 in]
        n446 = local write "VASPIFY Folder Name"(w753) -> ()
      }
      event "Show New Grain": Value Change {
        w833 = -0.01 ("norm")
        n447 = event-data() -> ()  [unwired: 1 in, 5 out]
        n448 = local read "Last Structures"() -> (w819:T1)
        n449 = Index Array(array=w819) -> (element=w818:T3)  [unwired: 1 in]
        n450 = Unbundle By Name(w818) -> ("Lattice vector a"=w826:dbl[], "Lattice vector b"=w825:dbl[], "Lattice vector c"=w824:dbl[], "Atoms Array"=w822:T20, "# of atoms"=w821:i32)
        n451 = disable-structure shown="Disabled" {
          disable-tunnel: w822 -> [w844 _]
          disable-tunnel: w821 -> [w841 _]
          disable-tunnel: [w840 w852] -> w820
          disable-tunnel: w818 -> [_ w858]
          frame Disabled {
            n452 = for {
              tunnel: w844 -> [w848] mode=indexing
              shift-right: [w846] -> w842
              shift-left: dbl[] [0.0, 0.0, 0.0] -> [w845]
              n453 = Unbundle By Name(w848) -> ("Positions (Cartesian)"=w847:dbl[][])
              n454 = for {
                tunnel: w847 -> [w851] mode=indexing
                shift-right: [w850] -> w846
                shift-left: w845 -> [w849]
                n455 = Add(x=w849, y=w851) -> (x+y=w850:dbl[])
              }
            }
            n456 = Divide(x=w842, y=w841) -> (x/y=w840:dbl[])
          }
          frame Enabled {
            n457 = Unbundle By Name(w858) -> ("Lattice vector a"=w857:dbl[], "Lattice vector b"=w856:dbl[], "Lattice vector c"=w855:dbl[])
            n458 = Compound Arithmetic op=ADD(w857, w856, w855) -> (w853:dbl[])
            n459 = Divide(x=w853, y=2.0) -> (x/y=w852:dbl[])
          }
        }
        n460 = call-poly <vilib>:"Vector Norm.vi"("Input Vector"=w826) -> ("norm"=w836:dbl)  [unwired: 9 in, 1 out]
        n461 = call-poly <vilib>:"Vector Norm.vi"("Input Vector"=w825) -> ("norm"=w835:dbl)  [unwired: 9 in, 1 out]
        n462 = call-poly <vilib>:"Vector Norm.vi"("Input Vector"=w824) -> ("norm"=w834:dbl)  [unwired: 9 in, 1 out]
        n463 = Bundle("norm"=w833, "norm"=w836, "norm"=w833, "norm"=w835, "norm"=w833, "norm"=w834) -> (w830:T21)  [unwired: 1 in]
        n464 = call "Find Subcrystal.vi"("Base Atom"="Base Atom", "Atomic Structure"=w818) -> ("Base Atom Position (Cartesian)"=w823:dbl[], "Subcrystal"=w838:T3)  [unwired: 7 in, 1 out]
        n465 = call "Translate Structure.vi"("Translation Vector (Cartesian)"=w823, "Atomic Structure"=w838) -> ("Shifted Structure"=w828:T3)  [unwired: 9 in]
        "GB Subcrystal" <- w828
        n466 = Multiply(x=w830, y=1.01 ("norm")) -> (x*y=w829:T21)
        n467 = call "Supercell Structure into a Box.vi"("Center Subcrystal"=FALSE, "Draw Box"=w829, "Subcrystal"=w828) -> ("Expanded cubic Structure"=w831:T3)  [unwired: 6 in, 2 out]
        n468 = call "Merge Two Structures (Cuboid).vi"("Translation Vector (1 to 2)"=w824, "Atomic Structure 2"=w831, "Atomic Structure 1"=w818) -> ("Atomic Structure of 1 + 2 by T"=w832:T3)  [unwired: 8 in]
        n469 = property on="Current Atomic Structure" class="Clust (strict)"("Val(Sgnl)"=w832) -> ()  [unwired: 2 in, 2 out]
        n470 = local write "Rotation Axis Intersection"(w820) -> ()
      }
      event "Suggest Draw Box": Value Change {
        w874 = 0.0 ("norm")
        n471 = event-data() -> ()  [unwired: 1 in, 5 out]
        n472 = local read "Last Structures"() -> (w860:T1)
        n473 = Index Array(array=w860) -> (element=w859:T3)  [unwired: 1 in]
        n474 = Unbundle By Name(w859) -> ("Lattice vector a"=w879:dbl[], "Lattice vector b"=w878:dbl[], "Lattice vector c"=w873:dbl[])
        n475 = call-poly <vilib>:"Vector Norm.vi"("Input Vector"=w879) -> ("norm"=w877:dbl)  [unwired: 9 in, 1 out]
        n476 = call-poly <vilib>:"Vector Norm.vi"("Input Vector"=w878) -> ("norm"=w876:dbl)  [unwired: 9 in, 1 out]
        n477 = call-poly <vilib>:"Vector Norm.vi"("Input Vector"=w873) -> ("norm"=w875:dbl)  [unwired: 9 in, 1 out]
        n478 = Bundle("norm"=w874, "norm"=w877, "norm"=w874, "norm"=w876, "norm"=w874, "norm"=w875) -> (w872:T21)  [unwired: 1 in]
        n479 = Multiply(x=w872, y=1.0 ("norm")) -> (x*y=w870:T21)
        n480 = Unbundle(w870) -> ("norm"=w869:dbl, "norm"=w868:dbl, "norm"=w867:dbl, "norm"=w866:dbl, "norm"=w865:dbl, "norm"=w864:dbl)
        n481 = Bundle("norm"=w869, "norm"=w868) -> (w863:cluster{"norm":dbl, "norm":dbl})  [unwired: 1 in]
        n482 = Bundle("norm"=w867, "norm"=w866) -> (w862:cluster{"norm":dbl, "norm":dbl})  [unwired: 1 in]
        n483 = Bundle("norm"=w865, "norm"=w864) -> (w861:cluster{"norm":dbl, "norm":dbl})  [unwired: 1 in]
        n484 = local write "GB Draw Box Y"(w862) -> ()
        n485 = local write "GB Draw Box X"(w863) -> ()
        n486 = local write "GB Draw Box Z"(w861) -> ()
      }
      event "Tilt Angle", "Twist Angle", "GB Draw Box X", "GB Draw Box Y", "GB Draw Box Z": Value Change {
        n487 = event-data() -> ()  [unwired: 1 in, 5 out]
        n488 = local read "Last Structures"() -> (w881:T1)
        n489 = Index Array(array=w881) -> (element=w880:T3)  [unwired: 1 in]
        n490 = local read "GB Subcrystal"() -> (w893:T3)
        n491 = Unbundle("GB Draw Box X") -> (w886:dbl, w887:dbl)
        n492 = Unbundle("GB Draw Box Y") -> (w888:dbl, w889:dbl)
        n493 = Unbundle("GB Draw Box Z") -> (w890:dbl, w891:dbl)
        n494 = call "Rotate Structure.vi"("Rotation Axis Intersection"="Rotation Axis Intersection", "Rotation Axis Direction"=dbl[] [1.0, 0.0, 0.0] ("Rotation Axis"), "Rotation Angle (Degree)"="Tilt Angle", "Atomic Structure"=w893) -> ("Rotated Sturcutre"=w899:T3)  [unwired: 7 in]
        n495 = Bundle(w886, w887, w888, w889, w890, w891) -> (w895:cluster{dbl, dbl, dbl, dbl, dbl, dbl})  [unwired: 1 in]
        n496 = Unbundle By Name(w880) -> ("Lattice vector c"=w892:dbl[])
        n497 = call "Rotate Structure.vi"("Rotation Axis Intersection"="Rotation Axis Intersection", "Rotation Axis Direction"=dbl[] [0.0, 0.0, 1.0] ("Rotation Axis"), "Rotation Angle (Degree)"="Twist Angle", "Atomic Structure"=w899) -> ("Rotated Sturcutre"=w896:T3)  [unwired: 7 in]
        n498 = call "Supercell Structure into a Box.vi"("Keep old lattice vectors?"=FALSE, "Center Subcrystal"=FALSE, "Draw Box"=w895, "Subcrystal"=w896) -> ("Expanded cubic Structure"=w902:T3)  [unwired: 5 in, 2 out]
        n499 = call "Merge Two Structures (Cuboid).vi"("Translation Vector (1 to 2)"=w892, "Atomic Structure 2"=w902, "Atomic Structure 1"=w880) -> ("Atomic Structure of 1 + 2 by T"=w903:T3)  [unwired: 8 in]
        n500 = property on="Current Atomic Structure" class="Clust (strict)"("Val(Sgnl)"=w903) -> ()  [unwired: 2 in, 2 out]
      }
      event "Atom List": Value Change {
        n501 = event-data() -> ()  [unwired: 1 in, 5 out]
        n502 = Empty Array?(array="Atom List") -> (empty?=w905:bool)
        n503 = case shown="True" "Highlight During Selection?" {
          tunnel: "Atom List" -> [_ w920]
          tunnel: w905 -> [_ w910]
          frame False {
          }
          frame True {
            n504 = local read "Base Object"() -> (w909:refnum<vi>)
            n505 = local read "Current Atomic Structure"() -> (w913:T3)
            n506 = local read "Atom Size"() -> (w915:dbl)
            n507 = Close Reference(reference=w909) -> (error out=w908:errorcluster)  [unwired: 1 in]
            n508 = local read "Options"() -> (w914:cluster{"Border?":bool, "Bonds?":bool})
            n509 = local read "Scale"() -> (w916:dbl)
            n510 = call <vilib>:"Create Object.vi"("error in (no error)"=w908, "Name"="Base") -> ("Scene:New Object"=w911:refnum<vi>)  [unwired: 9 out]
            n511 = Multiply(x=w916, y=w915) -> (x*y=w919:dbl)
            n512 = call "Render Structure.vi"("Options"=w914, "Atom Size"=w915, "Scale"=w916, "Atomic Structure"=w913, "Base Object"=w911) -> ("Object with atoms"=w917:refnum<vi>)  [unwired: 6 in]
            n513 = local write "Base Object"(w911) -> ()
            n514 = case shown="False" w910 {
              tunnel: w920 -> [w924 _]
              tunnel: w919 -> [w923 _]
              tunnel: [w922 w933] -> w918
              tunnel: w917 -> [w921 w933]
              frame False {
                n515 = for {
                  tunnel: w924 -> [w932] mode=indexing
                  tunnel: w923 -> [w927]
                  tunnel: [w926] -> w922
                  tunnel: w921 -> [w925]
                  n516 = call <vilib>:"Color Change.vi"("Color"="Highlight Color") -> ("RGBA"=w929:cluster{"R":sgl, "G":sgl, "B":sgl, "A":sgl})  [unwired: 10 in]
                  n517 = invoke class="SceneObject" method="Object.Get Object"(reference=w925, "Child Number"=w932) -> (reference out=w926:refnum<vi>, "Get Child"=w931:refnum<vi>)  [unwired: 2 in, 2 out]
                  n518 = call <vilib>:"Create Sphere.vi"("Color"=w929, "Radius"=w927) -> ("New Sphere Refnum"=w930:refnum<vi>)  [unwired: 8 in, 1 out]
                  n519 = invoke class="SceneObject" method="Set Drawable"(reference=w931, "Drawable"=w930) -> ()  [unwired: 2 in, 4 out]
                }
              }
              frame True {
              }
            }
            n520 = local write "Scene Display"(w918) -> ()
          }
        }
      }
      event "Periodicity", "Additional Strain/twin (A)", "Predict Best Strain": Value Change {
        n521 = event-data() -> ()  [unwired: 1 in, 5 out]
        n522 = Add Array Elements(numeric array="Periodicity") -> (sum=w952:i32)
        n523 = case shown="False" "Predict Best Strain" {
          tunnel: ["Additional Strain/twin (A)" w972] -> w938
          tunnel: w952 -> [_ w975]
          frame False {
          }
          frame True {
            n524 = Multiply(x=w975, y=0.0176338888888889 ("x")) -> (x*y=w973:dbl)
            n525 = Add(x=0.0449710222222222, y=w973) -> (x+y=w972:dbl)
            n526 = local write "Additional Strain/twin (A)"(w972) -> ()
          }
        }
        n527 = call "Create Arbitrary 111 Twin.vi"("Additional Strain/twin (A)"=w938, "Periodicity"="Periodicity") -> ("# of extra cells needed for cubic"=w944:i32, "AnBm Twin"=w946:T3)  [unwired: 8 in]
        "# of extra cells needed for cubic" <- w944
        n528 = property on="Current Atomic Structure" class="Clust (strict)"("Val(Sgnl)"=w946) -> ()  [unwired: 2 in, 2 out]
        n529 = Increment(x=w944) -> (x+1=w937:i32)
        n530 = Multiply(x=w938, y=w937) -> (x*y=w936:dbl)
        n531 = Multiply(x=w937, y=2) -> (x*y=w939:i32)
        n532 = Unbundle By Name(w946) -> ("Structure Name"=w945:string)
        n533 = Build Array (concatenate)(w939, w936, "Periodicity") -> (w942:dbl[])
        n534 = Number To Fractional String(number=w942) -> (F-format string=w941:string[])  [unwired: 3 in]
        n535 = Build Array (concatenate)(w945, w941) -> (w940:string[])
        n536 = local read "Headers"() -> (w950:string[])
        n537 = local read "Values"() -> (w949:string[])
        n538 = for {
          tunnel: string[] ["GB Name", "Number of Interfaces", "Strain (A)", "# of Bulk Columns (n)", "# of Twinned Columns (m)"] -> [w955] mode=indexing
          shift-right: [w956] -> w948
          shift-left: w950 -> [w957]
          shift-right: [w953] -> w947
          shift-left: w949 -> [w958]
          tunnel: w940 -> [w954] mode=indexing
          n539 = Search 1D Array(1D array=w957, element=w955) -> (index of element=w959:i32)  [unwired: 1 in]
          n540 = case shown="-1" w959 {
            selector: w959 -> [w963 _]
            tunnel: w958 -> [w964 w967]
            tunnel: [w962 w965] -> w953
            tunnel: w957 -> [w961 w970]
            tunnel: [w961 w968] -> w956
            tunnel: w955 -> [_ w969]
            tunnel: w954 -> [w960 w966]
            frame Default {
              n541 = Replace Array Subset(array=w964, new element=w960, index=w963) -> (w962:string[])
            }
            frame -1 {
              n542 = Build Array (concatenate)(w967, w966) -> (w965:string[])
              n543 = Build Array (concatenate)(w970, w969) -> (w968:string[])
            }
          }
        }
        n544 = local write "Headers"(w948) -> ()
        n545 = local write "Values"(w947) -> ()
      }
      event "Scene Display": Mouse Down {
        n546 = event-data() -> ("Coords"=w981:T24, "PlatMods"=w978:T27)  [unwired: 1 in, 5 out]
        n547 = property on="Scene Display" class="SceneGraphDisp (strict)"() -> ("Position"=w980:T28)  [unwired: 2 in, 2 out]
        n548 = Unbundle By Name(w978) -> ("Ctrl"=w977:bool)
        n549 = Subtract(x=w981, y=w980) -> (x-y=w979:T24)
        n550 = case shown="True" w977 {
          tunnel: w979 -> [_ w985]
          tunnel: w978 -> [_ w982]
          frame False {
          }
          frame True {
            n551 = invoke on="Scene Display" class="SceneGraphDisp (strict)" method="PickPoint"("PickPoint"=w985) -> ("PickPoint"=→"PickPoint":T2, "Hit"=w984:bool)  [unwired: 4 in, 3 out]
            n552 = case shown="True" w984 {
              tunnel: w985 -> [_ w1000]
              tunnel: w982 -> [_ w989]
              frame False {
              }
              frame True {
                n553 = invoke on="Scene Display" class="SceneGraphDisp (strict)" method="Pick Model"("Point"=w1000) -> ("Pick Model"=w999:cluster{"Node Path":refnum<vi>[]}[])  [unwired: 3 in, 3 out]
                n554 = Unbundle By Name(w989) -> ("Shift"=w988:bool)
                n555 = Index Array(array=w999) -> (element=w998:cluster{"Node Path":refnum<vi>[]})  [unwired: 1 in]
                n556 = Unbundle By Name(w998) -> ("Node Path"=w996:refnum<vi>[])
                n557 = Array Size(array=w996) -> (size(s)=w997:i32)
                n558 = Decrement(x=w997) -> (x-1=w995:i32)
                n559 = local read "Base Object"() -> (w993:refnum<vi>)
                n560 = Index Array(array=w996, index=w995) -> (element=w994:refnum<vi>)
                n561 = invoke class="SceneObject" method="Object.Object Count"(reference=w993) -> (reference out=w991:refnum<vi>, "Child Count"=w992:i32)  [unwired: 2 in, 1 out]
                n562 = property class="SceneObject"(reference=w994) -> ("Name"=w990:string)  [unwired: 1 in, 2 out]
                n563 = for {
                  N: w992 -> [_]
                  shift-right: [w1016] -> _
                  shift-left: w991 -> [w1017]
                  tunnel: w990 -> [w1012]
                  tunnel: [w1011] -> w987
                  i -> [w1011]
                  stop <- w1014 stop-if-true
                  n564 = invoke class="SceneObject" method="Object.Get Object"(reference=w1017, "Child Number"=w1011) -> (reference out=w1016:refnum<vi>, "Get Child"=w1015:refnum<vi>)  [unwired: 2 in, 2 out]
                  n565 = property class="SceneObject"(reference=w1015) -> ("Name"=w1013:string)  [unwired: 1 in, 2 out]
                  n566 = Equal?(x=w1013, y=w1012) -> (x = y?=w1014:bool)
                }
                n567 = case shown="True" w988 {
                  tunnel: w987 -> [w1002 w1004]
                  tunnel: [w1001 w1006] -> w986
                  frame False {
                    n568 = Build Array(w1002) -> (w1001:i32[])
